vi "InputPulseTriggeredOutput_V3_20250127.vi"() -> ()   [LabVIEW 2024]
uses:
  <vilib>/DAQmx/read.llb/DAQmx Read (Analog Wfm 1Chan 1Samp).vi
  <vilib>/DAQmx/write.llb/DAQmx Write (Analog Wfm 1Chan NSamp).vi
  <vilib>/DAQmx/create/channels.llb/DAQmx Create Channel (AI-Voltage-Basic).vi
  <vilib>/DAQmx/configure/timing.llb/DAQmx Timing (Sample Clock).vi
  <vilib>/DAQmx/create/channels.llb/DAQmx Create Channel (AO-Voltage-Basic).vi
  <vilib>/DAQmx/miscellaneous.llb/DAQmx Fill In Error Info.vi
  <vilib>/measure/mamon.llb/Trigger Detection for 1 Channel.vi
  <vilib>/measure/NI_MAPro.lvlib
panel:
  in  "Time Between Stimulation (s)":dbl=5.0 min=5.0 max=200.0 step=1.0
  in  "Pulse Dur (ms)":dbl=1.0 min=1.0 max=1000.0 step=1.0
  in  "Pulse Gap (ms)":dbl=1.0 min=1.0 max=1000.0 step=1.0
  in  "Amp (mA)":dbl=0.1 min=0.1 max=50.0 step=0.1
  in  "Pulse Repeats":dbl=1.0 min=1.0 max=1000.0 step=1.0
  out "Stimulation Parameters":picture
  out "Overview":picture
  out "data":waveform(dbl)
  in  "stop 2":bool
  in  "stop":bool
  out "trigger detected?":bool
  out "previous stim value":bool
  in  "STIM":bool
  out "Read from DAQ":waveform(dbl)(graph)
  in  "Pulse width 1 (ms)":dbl=1.0 format="%0.2f"
  in  "Frequency (Hz)":dbl=1.0 format="%0.2p"
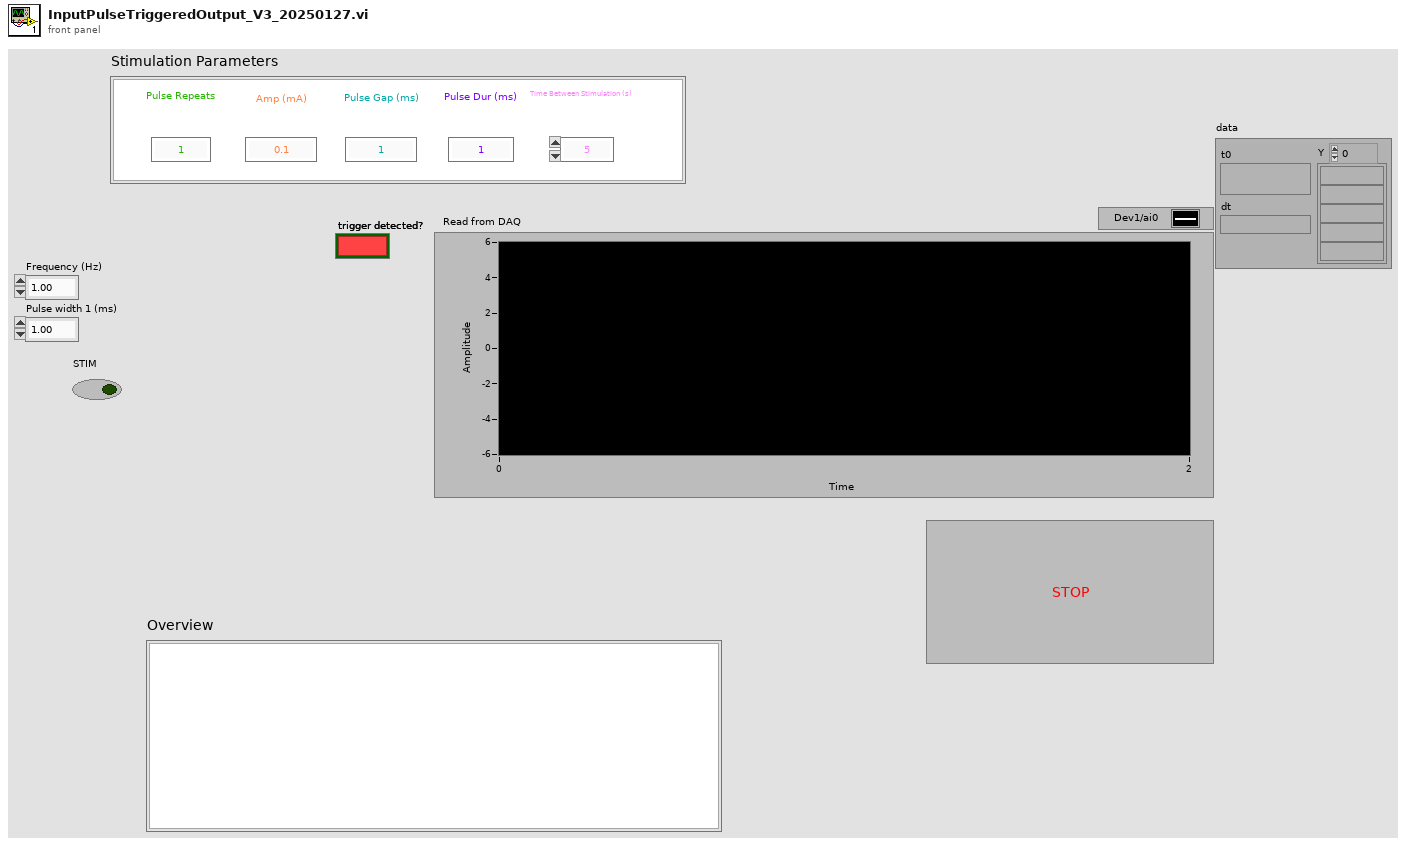
[diagram p1: front panel]
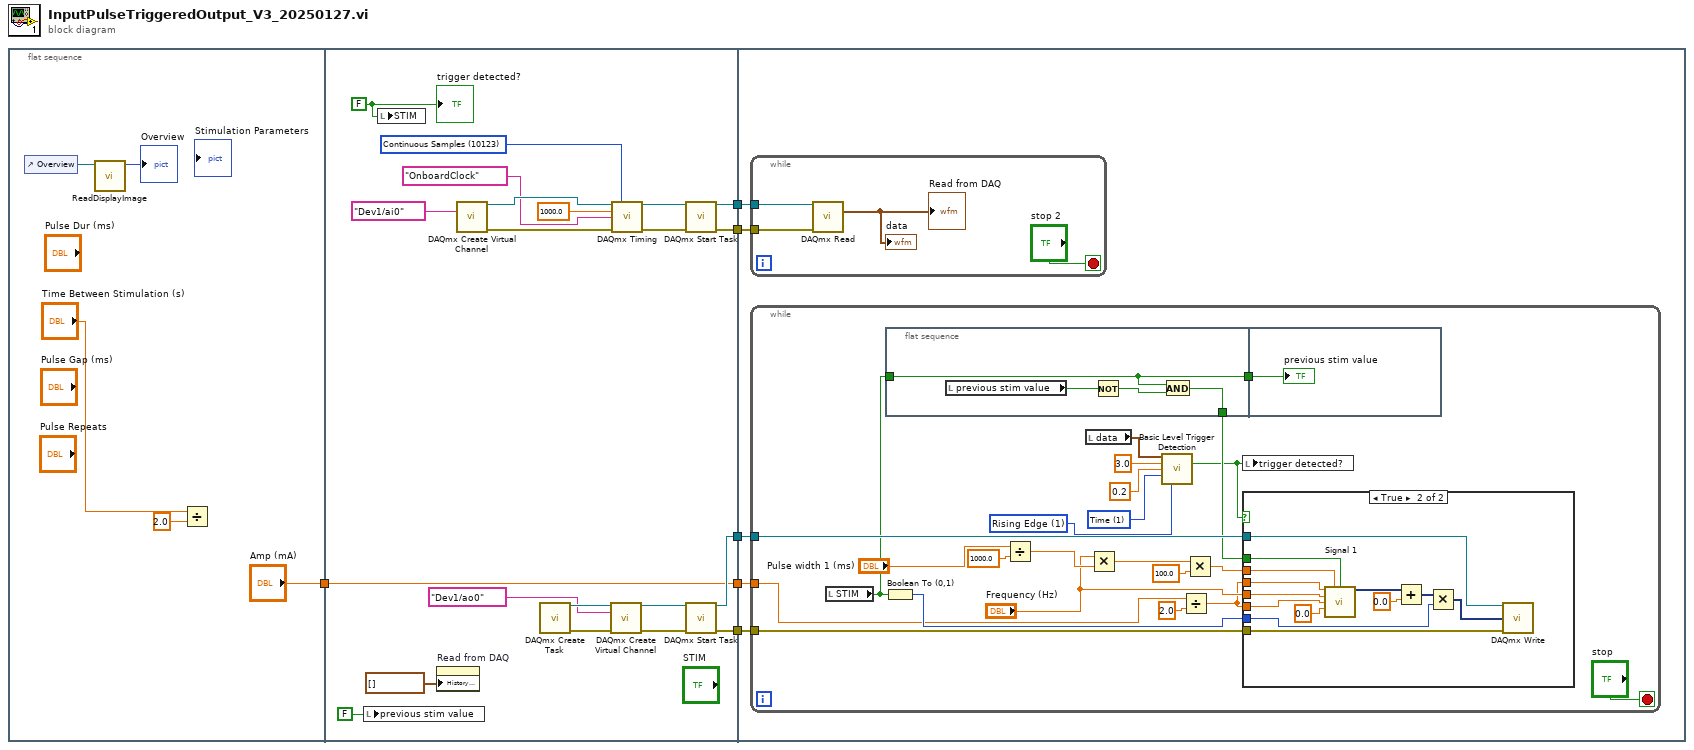
[diagram p0: block diagram]
diagram:
  n1 = flat-sequence {
    tunnel: ["Amp (mA)"] -> w2
    tunnel: [w18] -> w6
    tunnel: [w17] -> w5
    tunnel: [w16] -> w4
    tunnel: [w15] -> w3
    tunnel: w2 -> [w12]
    tunnel: [w12] -> w1
    tunnel: w6 -> [w37]
    tunnel: w5 -> [w36]
    tunnel: w4 -> [w35]
    tunnel: w3 -> [w34]
    tunnel: w1 -> [w33]
    frame #0 {
      n2 = control-ref of="Overview"() -> (w10:refnum<vi>)
      n3 = call "ReadDisplayImage.vi"("Picture in"=w10) -> ("Overview"=→"Overview":picture)  [unwired: 10 in]
      n4 = Divide(x="Time Between Stimulation (s)", y=2.0) -> ()  [unwired: 1 out]
    }
    frame #1 {
      w14 = FALSE ("STIM")
      w23 = 10123 items=["Finite Samples"=10178, "Continuous Samples"=10123, "Hardware Timed Single Point"=12522] ("sample mode")
      n5 = local write "previous stim value"(FALSE ("previous stim value")) -> ()
      n6 = local write "STIM"(w14) -> ()
      n7 = property on="Read from DAQ" class="WFChart (strict)"("History Data"=waveform(dbl)[] []) -> ()  [unwired: 2 in, 2 out]
      n8 = call-poly <vilib>:"DAQmx Create Virtual Channel.vi"("physical channels"=tag "Dev1/ai0") -> ("task out"=w24:refnum<k21>, "error out"=w27:errorcluster)  [unwired: 13 in]
      n9 = call <vilib>:"DAQmx Create Task.vi"() -> ("task out"=w29:refnum<k21>, "error out"=w30:errorcluster)  [unwired: 14 in]
      n10 = call-poly <vilib>:"DAQmx Create Virtual Channel.vi"("task in"=w29, "physical channels"=tag "Dev1/ao0", "error in"=w30) -> ("task out"=w31:refnum<k21>, "error out"=w32:errorcluster)  [unwired: 11 in]
      n11 = call-poly <vilib>:"DAQmx Timing.vi"("task/channels in"=w24, "sample mode"=w23, "rate"=1000.0, "source"=tag "OnboardClock", "error in"=w27) -> ("task out"=w25:refnum<k21>, "error out"=w26:errorcluster)  [unwired: 9 in]
      n12 = call <vilib>:"DAQmx Start Task.vi"("task/channels in"=w25, "error in"=w26) -> ("task out"=w16:refnum<k21>, "error out"=w15:errorcluster)  [unwired: 12 in]
      n13 = call <vilib>:"DAQmx Start Task.vi"("task/channels in"=w31, "error in"=w32) -> ("task out"=w18:refnum<k21>, "error out"=w17:errorcluster)  [unwired: 12 in]
      "trigger detected?" <- w14
    }
    frame #2 {
      n14 = while {
        tunnel: w35 -> [w39]
        tunnel: w34 -> [w38]
        stop <- "stop 2" stop-if-true
        n15 = call-poly <vilib>:"DAQmx Read.vi"("task/channels in"=w39, "error in"=w38) -> ("data"=→"Read from DAQ" →"data":waveform(dbl))  [unwired: 11 in, 2 out]
      }
      n16 = while {
        tunnel: w37 -> [w53]
        tunnel: w36 -> [w52]
        tunnel: w33 -> [w42]
        stop <- "stop" stop-if-true
        w55 = u16 1 items=["Index", "Time"] ("location mode")
        w54 = u16 1 items=["Falling Edge", "Rising Edge"] ("trigger slope")
        n17 = local read "STIM"() -> (w45:bool)
        n18 = Boolean To (0,1)(Boolean=w45) -> (0, 1=w51:i16)
        n19 = flat-sequence {
          tunnel: [w79] -> w64
          tunnel: w45 -> [w79]
          tunnel: [w78] -> w49
          tunnel: w64 -> [w82]
          frame #0 {
            n20 = local read "previous stim value"() -> (w80:bool)
            n21 = Not(x=w80) -> (.not. x?=w81:bool)
            n22 = And(x=w79, y=w81) -> (x .and. y?=w78:bool)
          }
          frame #1 {
            "previous stim value" <- w82
          }
        }
        n23 = Divide(x="Pulse width 1 (ms)", y=1000.0) -> (x/y=w60:dbl)
        n24 = local read "data"() -> (w43:waveform(dbl))
        n25 = Multiply(x="Frequency (Hz)", y=w60) -> (x*y=w58:dbl)
        n26 = call-poly <vilib>:"Basic Level Trigger Detection.vi"("signal in"=w43, "level"=3.0, "hysteresis"=0.2, "location mode"=w55, "trigger slope"=w54) -> ("trigger detected?"=w46:bool)  [unwired: 8 in, 2 out]
        n27 = Divide(x=w42, y=2.0) -> (x/y=w47:dbl)
        n28 = Multiply(x=w58, y=100.0) -> (x*y=w50:dbl)
        n29 = local write "trigger detected?"(w46) -> ()
        n30 = case shown="True" w46 {
          tunnel: w53 -> [_ w74]
          tunnel: w52 -> [_ w73]
          tunnel: w51 -> [_ w71]
          tunnel: w47 -> [_ w70]
          tunnel: w50 -> [_ w69]
          tunnel: w49 -> [_ w68]
          tunnel: "Frequency (Hz)" -> [_ w67]
          tunnel: w47 -> [_ w66]
          frame False {
          }
          frame True {
            n31 = call "Signal 1"("Offset"=w70, "Duty Cycle (%)"=w69, "Reset Signal"=w68, "Frequency"=w67, "Amplitude"=w66, "Phase"=0.0) -> ("Square"=w75:dynamicdata)  [unwired: 8 in, 1 out]
            n32 = Add(x=w75, y=0.0) -> (x+y=w76:dynamicdata)
            n33 = Multiply(x=w76, y=w71) -> (x*y=w77:dynamicdata)
            n34 = call-poly <vilib>:"DAQmx Write.vi"("task/channels in"=w74, "data"=w77, "error in"=w73) -> ()  [unwired: 10 in, 3 out]
          }
        }
      }
    }
  }
